vi "Ex1_Add_NET_Array.vi"() -> ()   [LabVIEW 2013]
uses:
  Ex1_add/for_testing/Ex1_add.dll
  <vilib>/Analysis/2dsp.llb/Decimate (continuous, DBL).vi
  <vilib>/Analysis/NI_AALPro.lvlib
panel:
  out "Array_1":dbl[](array[numeric])
  out "ToString":string
  out "Array_2":dbl[](array[numeric])
  in  "b":dbl[](array[numeric])
  in  "a":dbl[](array[numeric])
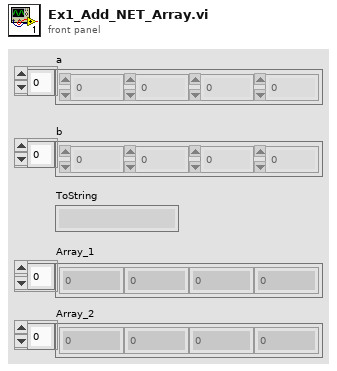
[diagram p1: front panel]
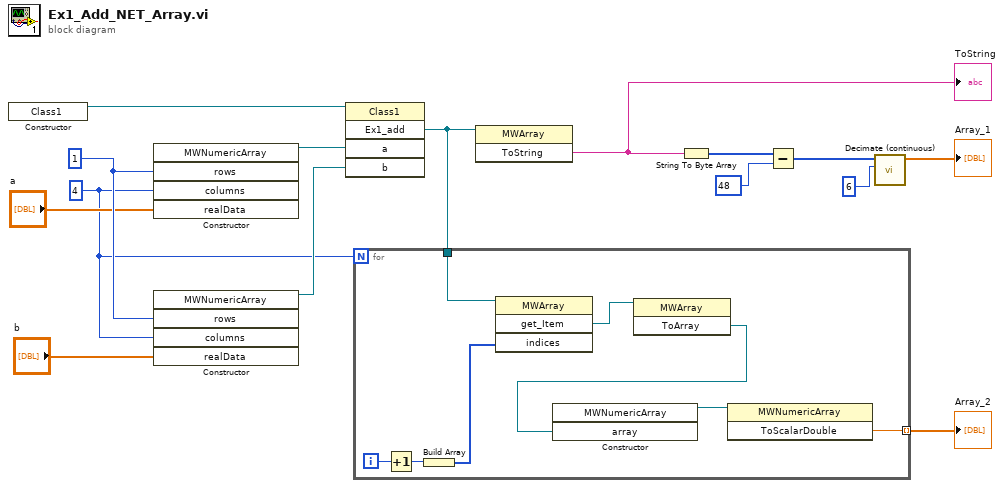
[diagram p0: block diagram]
diagram:
  w1 = 4 ("rows")
  w12 = 1 ("rows")
  n1 = constructor class="Class1"() -> (reference out=w15:refnum<k24>)  [unwired: 3 in, 2 out]
  n2 = constructor class="MWNumericArray"("rows"=w12, "columns"=w1, "realData"="a") -> (reference out=w14:refnum<k24>)  [unwired: 3 in, 5 out]
  n3 = constructor class="MWNumericArray"("rows"=w12, "columns"=w1, "realData"="b") -> (reference out=w13:refnum<k24>)  [unwired: 3 in, 5 out]
  n4 = invoke class="Class1" method="Ex1_add"(reference=w15, "a"=w14, "b"=w13) -> ("Ex1_add"=w8:refnum<k24>)  [unwired: 2 in, 4 out]
  n5 = for {
    N: w1 -> [_]
    tunnel: [w22] -> w9 mode=indexing
    tunnel: w8 -> [w21]
    i -> [w19]
    n6 = Increment(x=w19) -> (x+1=w18:i32)
    n7 = Build Array(w18) -> (w17:i32[])
    n8 = invoke class="MWArray" method="get_Item"(reference=w21, "indices"=w17) -> ("get_Item"=w20:refnum<k24>)  [unwired: 2 in, 3 out]
    n9 = invoke class="MWArray" method="ToArray"(reference=w20) -> ("ToArray"=w16:refnum<k24>)  [unwired: 2 in, 2 out]
    n10 = constructor class="MWNumericArray"("array"=w16) -> (reference out=w23:refnum<k24>)  [unwired: 3 in, 3 out]
    n11 = invoke class="MWNumericArray" method="ToScalarDouble"(reference=w23) -> ("ToScalarDouble"=w22:dbl)  [unwired: 2 in, 2 out]
  }
  "Array_2" <- w9
  n12 = invoke class="MWArray" method="ToString"(reference=w8) -> ("ToString"=w7:string)  [unwired: 2 in, 2 out]
  "ToString" <- w7
  n13 = String To Byte Array(string=w7) -> (unsigned byte array=w6:u8[])
  n14 = Subtract(x=w6, y=u8 48) -> (x-y=w2:u8[])
  n15 = call-poly <vilib>:"Decimate (continuous).vi"("decimating factor"=6, "X"=w2) -> ("Decimated Array"=→"Array_1":dbl[])  [unwired: 8 in, 1 out]
